vi "Read TestTeam.vi"(8 "error in (no error)":errorcluster, 11 "Game in":refnum<class "Game.lvclass">) -> (0 "error out":errorcluster, 2 "Ally":refnum<class "Ally.lvclass">, 3 "Game out":refnum<class "Game.lvclass">)   [LabVIEW 2020, in "Game.lvclass"]
uses:
  Game.lvclass
  Ally_class/Ally.lvclass
  Game.lvclass/Game.ctl
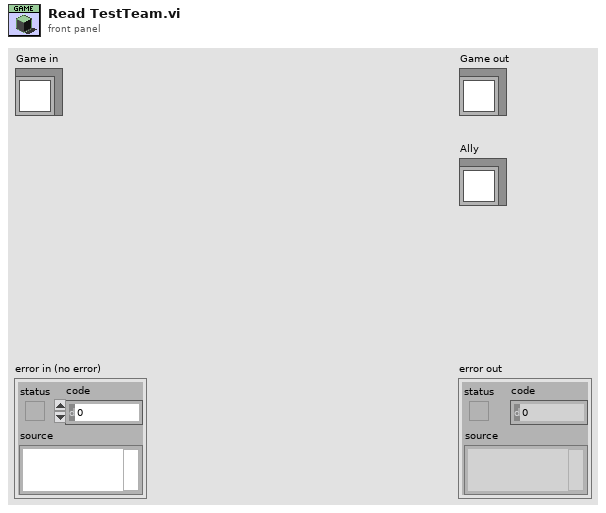
[diagram p1: front panel]
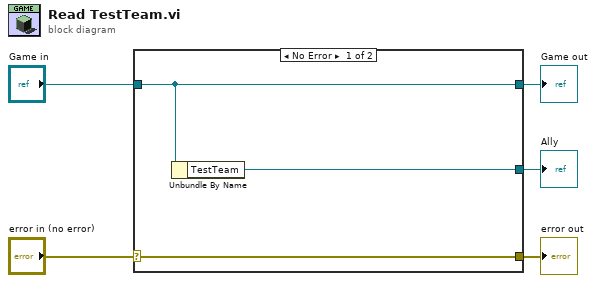
[diagram p0: block diagram]
diagram:
  n1 = case shown="No Error" "error in (no error)" {
    selector: "error in (no error)" -> [w8 w9]
    tunnel: [w8 w9] -> w4
    tunnel: [w7 w10] -> w2
    tunnel: "Game in" -> [w7 w10]
    tunnel: [w6 _] -> w1
    frame No Error {
      n2 = Unbundle By Name(w7) -> ("TestTeam"=w6:refnum<class "Ally.lvclass">)
    }
    frame Error {
    }
  }
  "error out" <- w4
  "Game out" <- w2
  "Ally" <- w1
